vi "Disabled - Message Delay (SubVI).vi"(10 "Time (s)":u32=3, 11 "Start Timer":bool) -> (3 "Timer's Up!":bool)   [LabVIEW 2015]
panel:
  # "Inputs"
  # "Outputs"
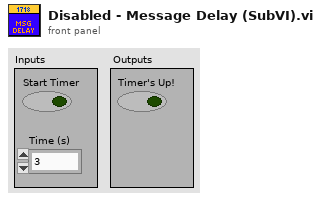
[diagram p1: front panel]
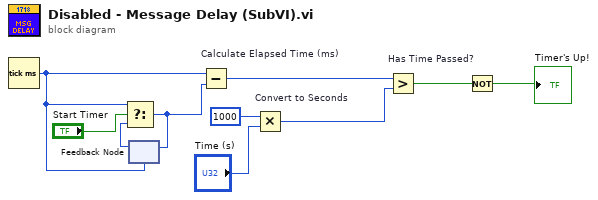
[diagram p0: block diagram]
diagram:
  n1 = Tick Count (ms)() -> (millisecond timer value=w7:u32)
  n2 = feedback #1(w7) -> (w2:u32)
  n3 = Select(t=w7, s="Start Timer", f=w2) -> (s? t:f=w3:u32)
  n4 = feedback-in #1(w3) -> ()
  n5 = Subtract "Calculate Elapsed Time (ms)"(x=w7, y=w3) -> (x-y=w4:u32)
  n6 = Multiply "Convert to Seconds"(x=u32 1000, y="Time (s)") -> (x*y=w10:u32)
  n7 = Greater? "Has Time Passed?"(x=w4, y=w10) -> (0:w5:bool)
  n8 = Not(x=w5) -> (.not. x?=→"Timer's Up!":bool)
